vi "GEOM_RCSimUseCols.vi"(9 "ROIS":T1(array[cluster]), 10 "amplifiers":T2[](array[typedef]) {"fliped" items=["none", "horizontal", "vertical"]; "type" items=["LL", "LR", "UL", "UR"]}) -> (1 "Corrected ROIs":T1(array[cluster]))   [LabVIEW 2016]
uses:
  GEOM_Amplifier.ctl
  GEOM_AmpType.ctl
  GEOM_ROI.ctl
  GEOM_Coords.ctl
panel:
  in  "Case Constant\n(See Context Help)":bool
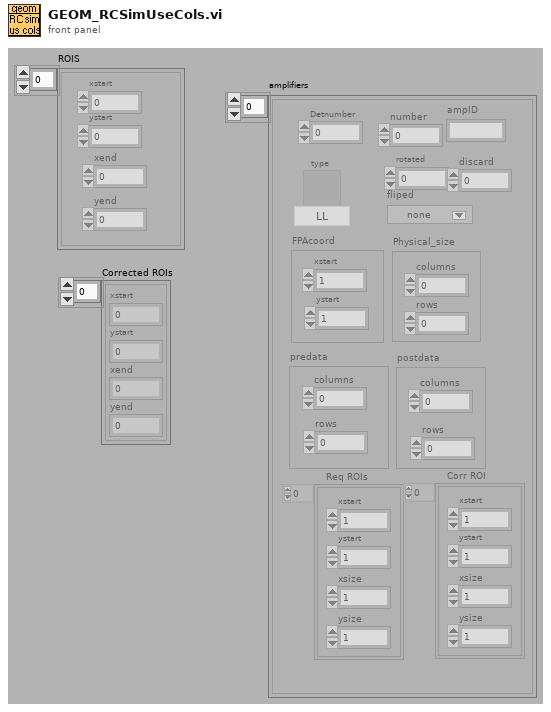
[diagram p1: front panel]
types:
  T1 = cluster{"xstart":i32, "ystart":i32, "xend":i32, "yend":i32}[]
  T2 = typedef "GEOM_Amplifier.ctl" = cluster{"number":i32, "type":T3, "rotated":i16, "fliped":u16, "FPAcoord":cluster{"xstart":i32, "ystart":i32}, "Physical_size":cluster{"columns":i32, "rows":i32}, "predata":cluster{"columns":i32, "rows":i32}, "postdata":cluster{"columns":i32, "rows":i32}, "Req ROIs":T4, "Corr ROI":T4, "Detnumber":i32, "ampID":string, "discard":i32}
  T3 = typedef "GEOM_AmpType.ctl" = u16
  T4 = typedef "GEOM_ROI.ctl" = T5[]
  T5 = typedef "GEOM_Coords.ctl" = cluster{"xstart":u32, "ystart":u32, "xsize":u32, "ysize":u32}
  T6 = cluster{"xstart":i32, "ystart":i32, "xend":i32, "yend":i32}
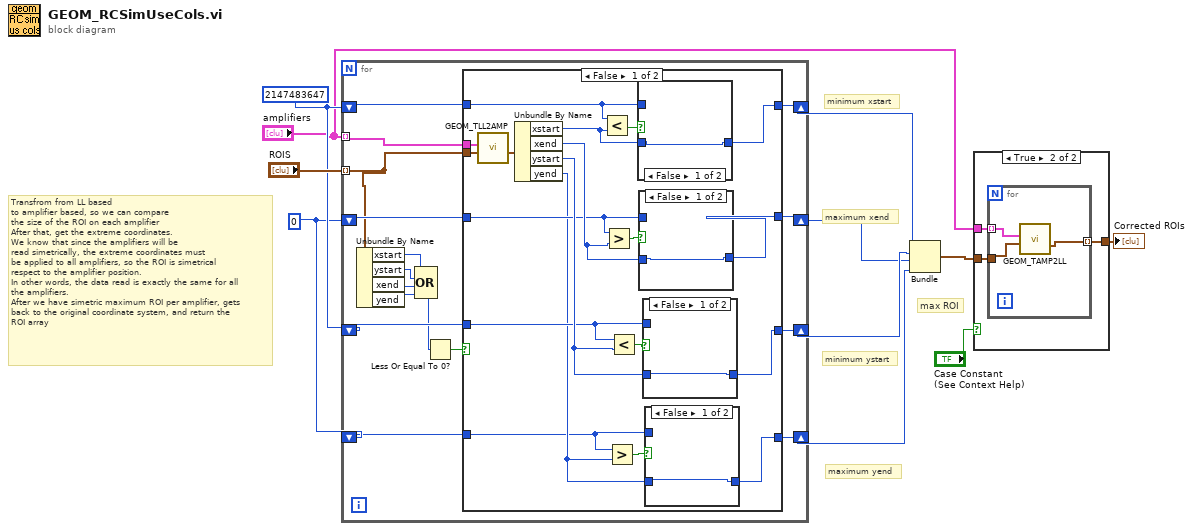
[diagram p0: block diagram]
diagram:
  w9 = 0
  w10 = 2147483647
  # "Transfrom from LL based\nto amplifier based, so we can compare\nthe size of the ROI on each amplifier\nAfter that, get the extreme coordinates.\nWe know that since the amplifiers will be \nread simetrically, the extreme coordinates must\nbe applied to all amplifiers, so the ROI is simetrical\nrespect to the amplifier position.\nIn other words, the data read is exactly the same for all\nthe amplifiers. \nAfter we have simetric maximum ROI per amplifier, gets\nback to the original coordinate system, and return the\nROI array"
  # "max ROI"
  # "maximum yend"
  # "minimum ystart"
  # "maximum xend"
  # "minimum xstart"
  n1 = for {
    tunnel: "ROIS" -> [w18] mode=indexing
    tunnel: "amplifiers" -> [w27] mode=indexing
    shift-right: [w26] -> w8
    shift-left: w10 -> [w25]
    shift-right: [w19] -> w6
    shift-left: w9 -> [w23]
    shift-right: [w24] -> w7
    shift-left: w10 -> [w22]
    shift-right: [w21] -> w5
    shift-left: w9 -> [w20]
    n2 = Unbundle By Name(w18) -> ("xstart"=w17:i32, "ystart"=w16:i32, "xend"=w15:i32, "yend"=w14:i32)
    n3 = Compound Arithmetic op=OR(w17, w16, w15, w14) -> (w13:i32)
    n4 = Less Or Equal To 0?(x=w13) -> (x <= 0?=w12:bool)
    n5 = case shown="False" w12 {
      tunnel: w27 -> [w46 _]
      tunnel: w18 -> [w45 _]
      tunnel: [w38 w58] -> w26
      tunnel: w25 -> [w37 w58]
      tunnel: [w34 w56] -> w24
      tunnel: w23 -> [w33 w57]
      tunnel: w22 -> [w32 w56]
      tunnel: [w30 w55] -> w21
      tunnel: w20 -> [w29 w55]
      tunnel: [w28 w57] -> w19
      frame False {
        n6 = call "GEOM_TLL2AMP.vi"("DETROIcoords"=w45, "Amplifier"=w46) -> ("AMPROICoords"=w44:T6)  [unwired: 9 out]
        n7 = Unbundle By Name(w44) -> ("xstart"=w42:i32, "xend"=w36:i32, "ystart"=w35:i32, "yend"=w31:i32)
        n8 = Less?(x=w37, y=w42) -> (x < y?=w43:bool)
        n9 = Greater?(x=w33, y=w36) -> (0:w40:bool)
        n10 = Greater?(x=w29, y=w31) -> (0:w41:bool)
        n11 = Less?(x=w32, y=w35) -> (x < y?=w39:bool)
        n12 = case shown="False" w43 {
          tunnel: w42 -> [w53 _]
          tunnel: [w53 w54] -> w38
          tunnel: w37 -> [_ w54]
          frame False {
          }
          frame True {
          }
        }
        n13 = case shown="False" w40 {
          tunnel: [w51 w52] -> w28
          tunnel: w36 -> [w51 _]
          tunnel: w33 -> [_ w52]
          frame False {
          }
          frame True {
          }
        }
        n14 = case shown="False" w39 {
          tunnel: w35 -> [w49 _]
          tunnel: [w49 w50] -> w34
          tunnel: w32 -> [_ w50]
          frame False {
          }
          frame True {
          }
        }
        n15 = case shown="False" w41 {
          tunnel: w31 -> [w47 _]
          tunnel: [w47 w48] -> w30
          tunnel: w29 -> [_ w48]
          frame False {
          }
          frame True {
          }
        }
      }
      frame True {
      }
    }
  }
  n16 = Bundle(w8, w7, w6, w5) -> (w4:cluster{i32, i32, i32, i32})  [unwired: 1 out]
  n17 = case shown="True" "Case Constant\n(See Context Help)" {
    tunnel: w4 -> [w60 w65]
    tunnel: "amplifiers" -> [w61 w64]
    tunnel: [w59 w63] -> w2
    frame False {
      n18 = for {
        tunnel: w61 -> [_] mode=indexing
        tunnel: w60 -> [w62]
        tunnel: [w62] -> w59 mode=indexing
      }
    }
    frame True {
      n19 = for {
        tunnel: w65 -> [w67]
        tunnel: w64 -> [w68] mode=indexing
        tunnel: [w66] -> w63 mode=indexing
        n20 = call "GEOM_TAMP2LL.vi"("AMPROIcoords"=w67, "Amplifier"=w68) -> ("DETROICoords"=w66:T6)  [unwired: 9 out]
      }
    }
  }
  "Corrected ROIs" <- w2
